vi "lijndetectie.vi"() -> ()   [LabVIEW 2019]
uses:
  <vilib>/Analysis/baseanly.llb/Real Dot Product.vi
  <vilib>/Analysis/NI_AALBase.lvlib
panel:
  out "?":i32
  out "motoren uit (stoppen)":bool
  out "motor links sneller 3":bool
  out "allebei even snel":bool
  out "motor rechts sneller":bool
  in  "input array":dbl[](array[numeric])
  in  "array 2":dbl[](array[numeric])
  out "array gelijk?":string="array gelijk"
  out "array gelijk?":bool[](array[boolean])
  out "true false output 2":bool[](array[boolean])
  out "true false output":bool[](array[boolean])
  out "aantal enen  instant":i32
  out "aantal enen":i32
  in  "array 1":dbl[](array[numeric])
  in  "Numeric 5":dbl
  out "Numeric 4":dbl
  in  "Numeric 2":dbl
  out "output array 2":i32[](array[numeric])
  out "output array":i32[](array[numeric])
  in  "Numeric 3":i32
  out "Numeric":i32
  out "dot product laatste 3 elmenten":dbl format="%.2f"
  out "X * Y":dbl format="%.2f"
  out "som":dbl
  out "x*y":dbl[](array[numeric])
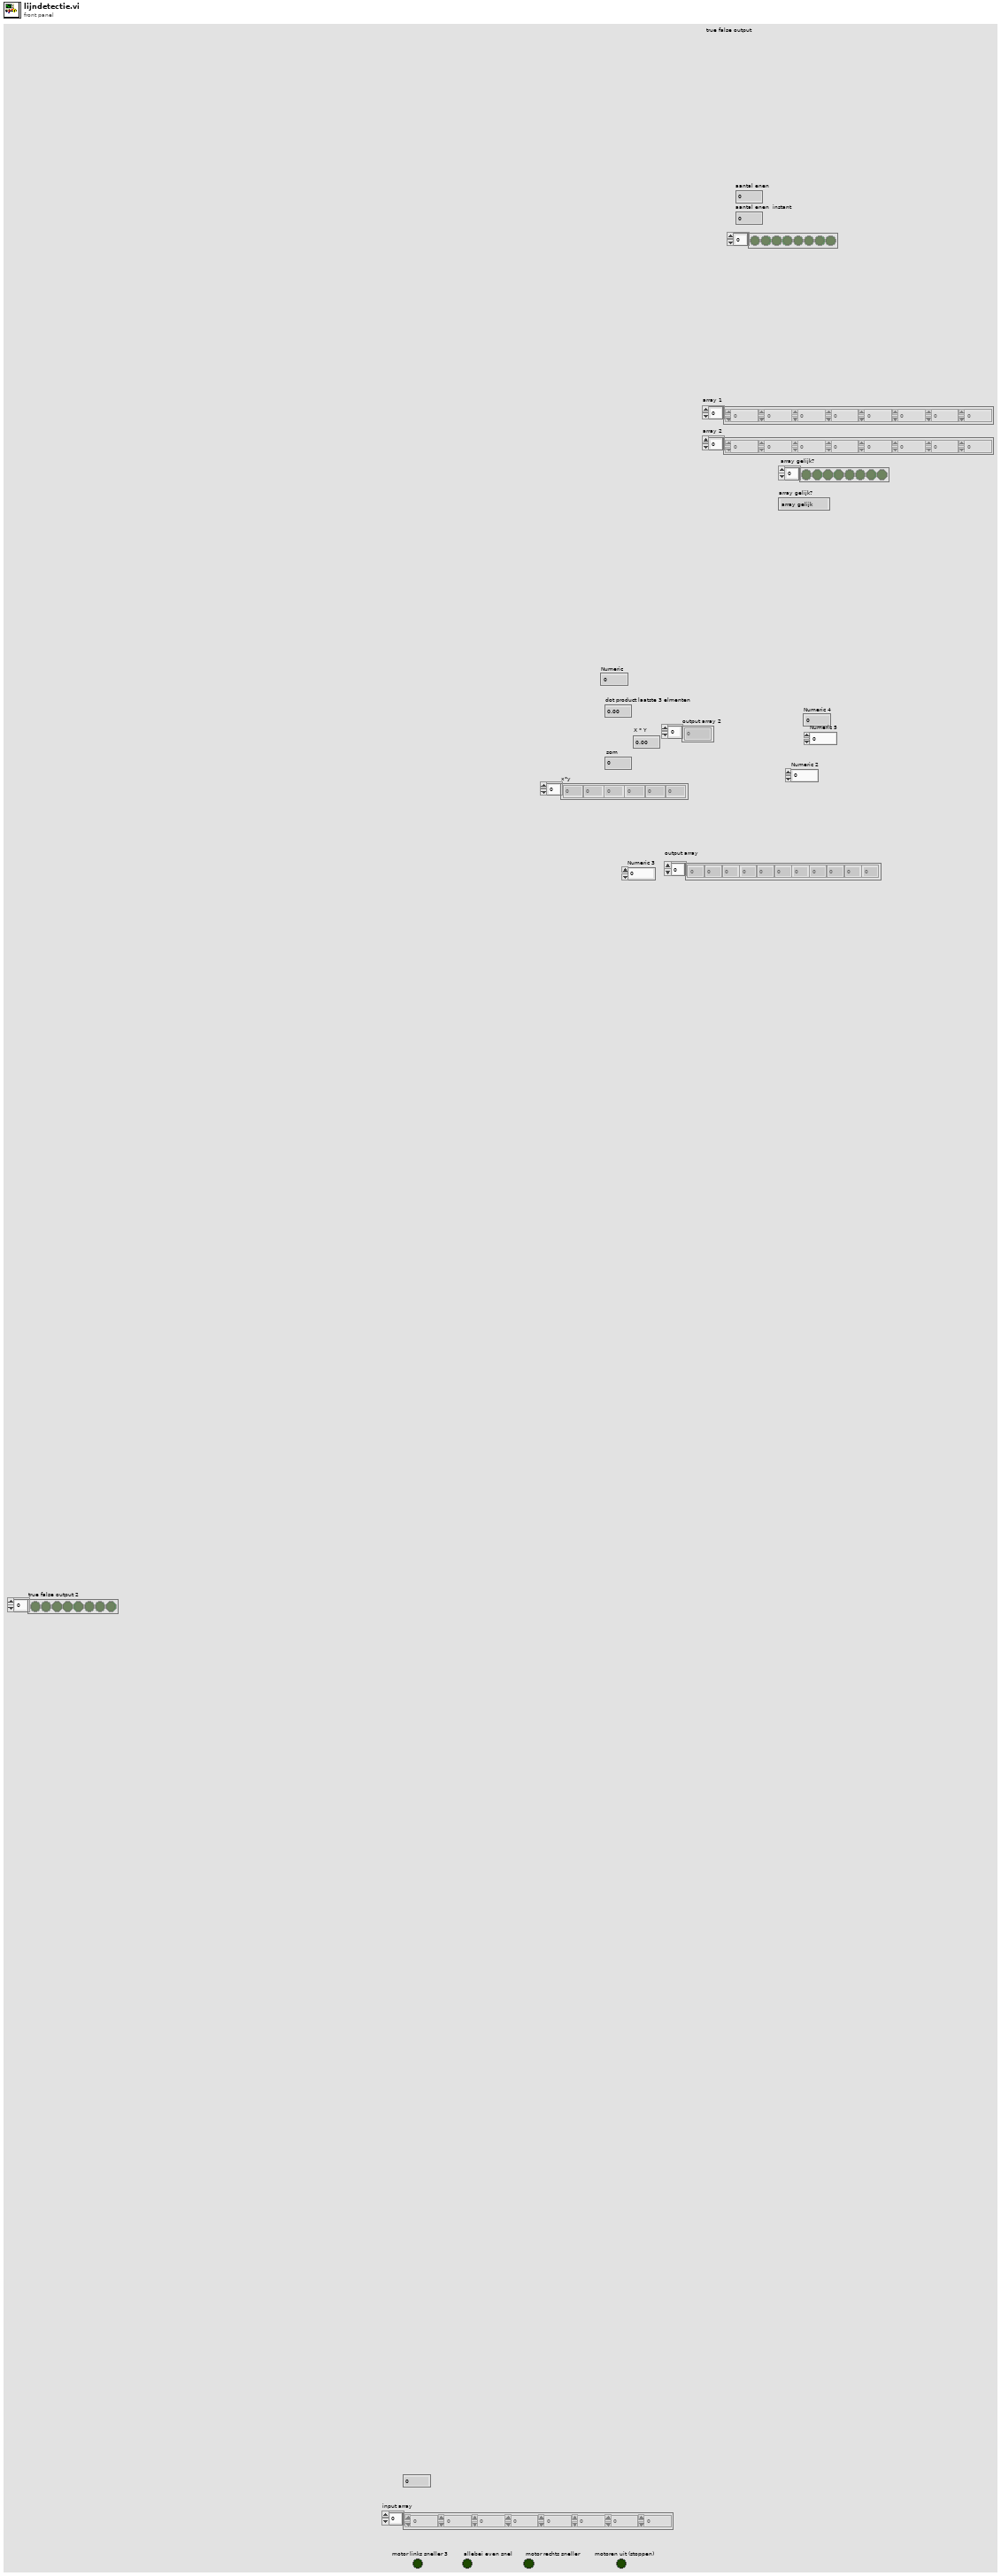
[diagram p1: front panel]
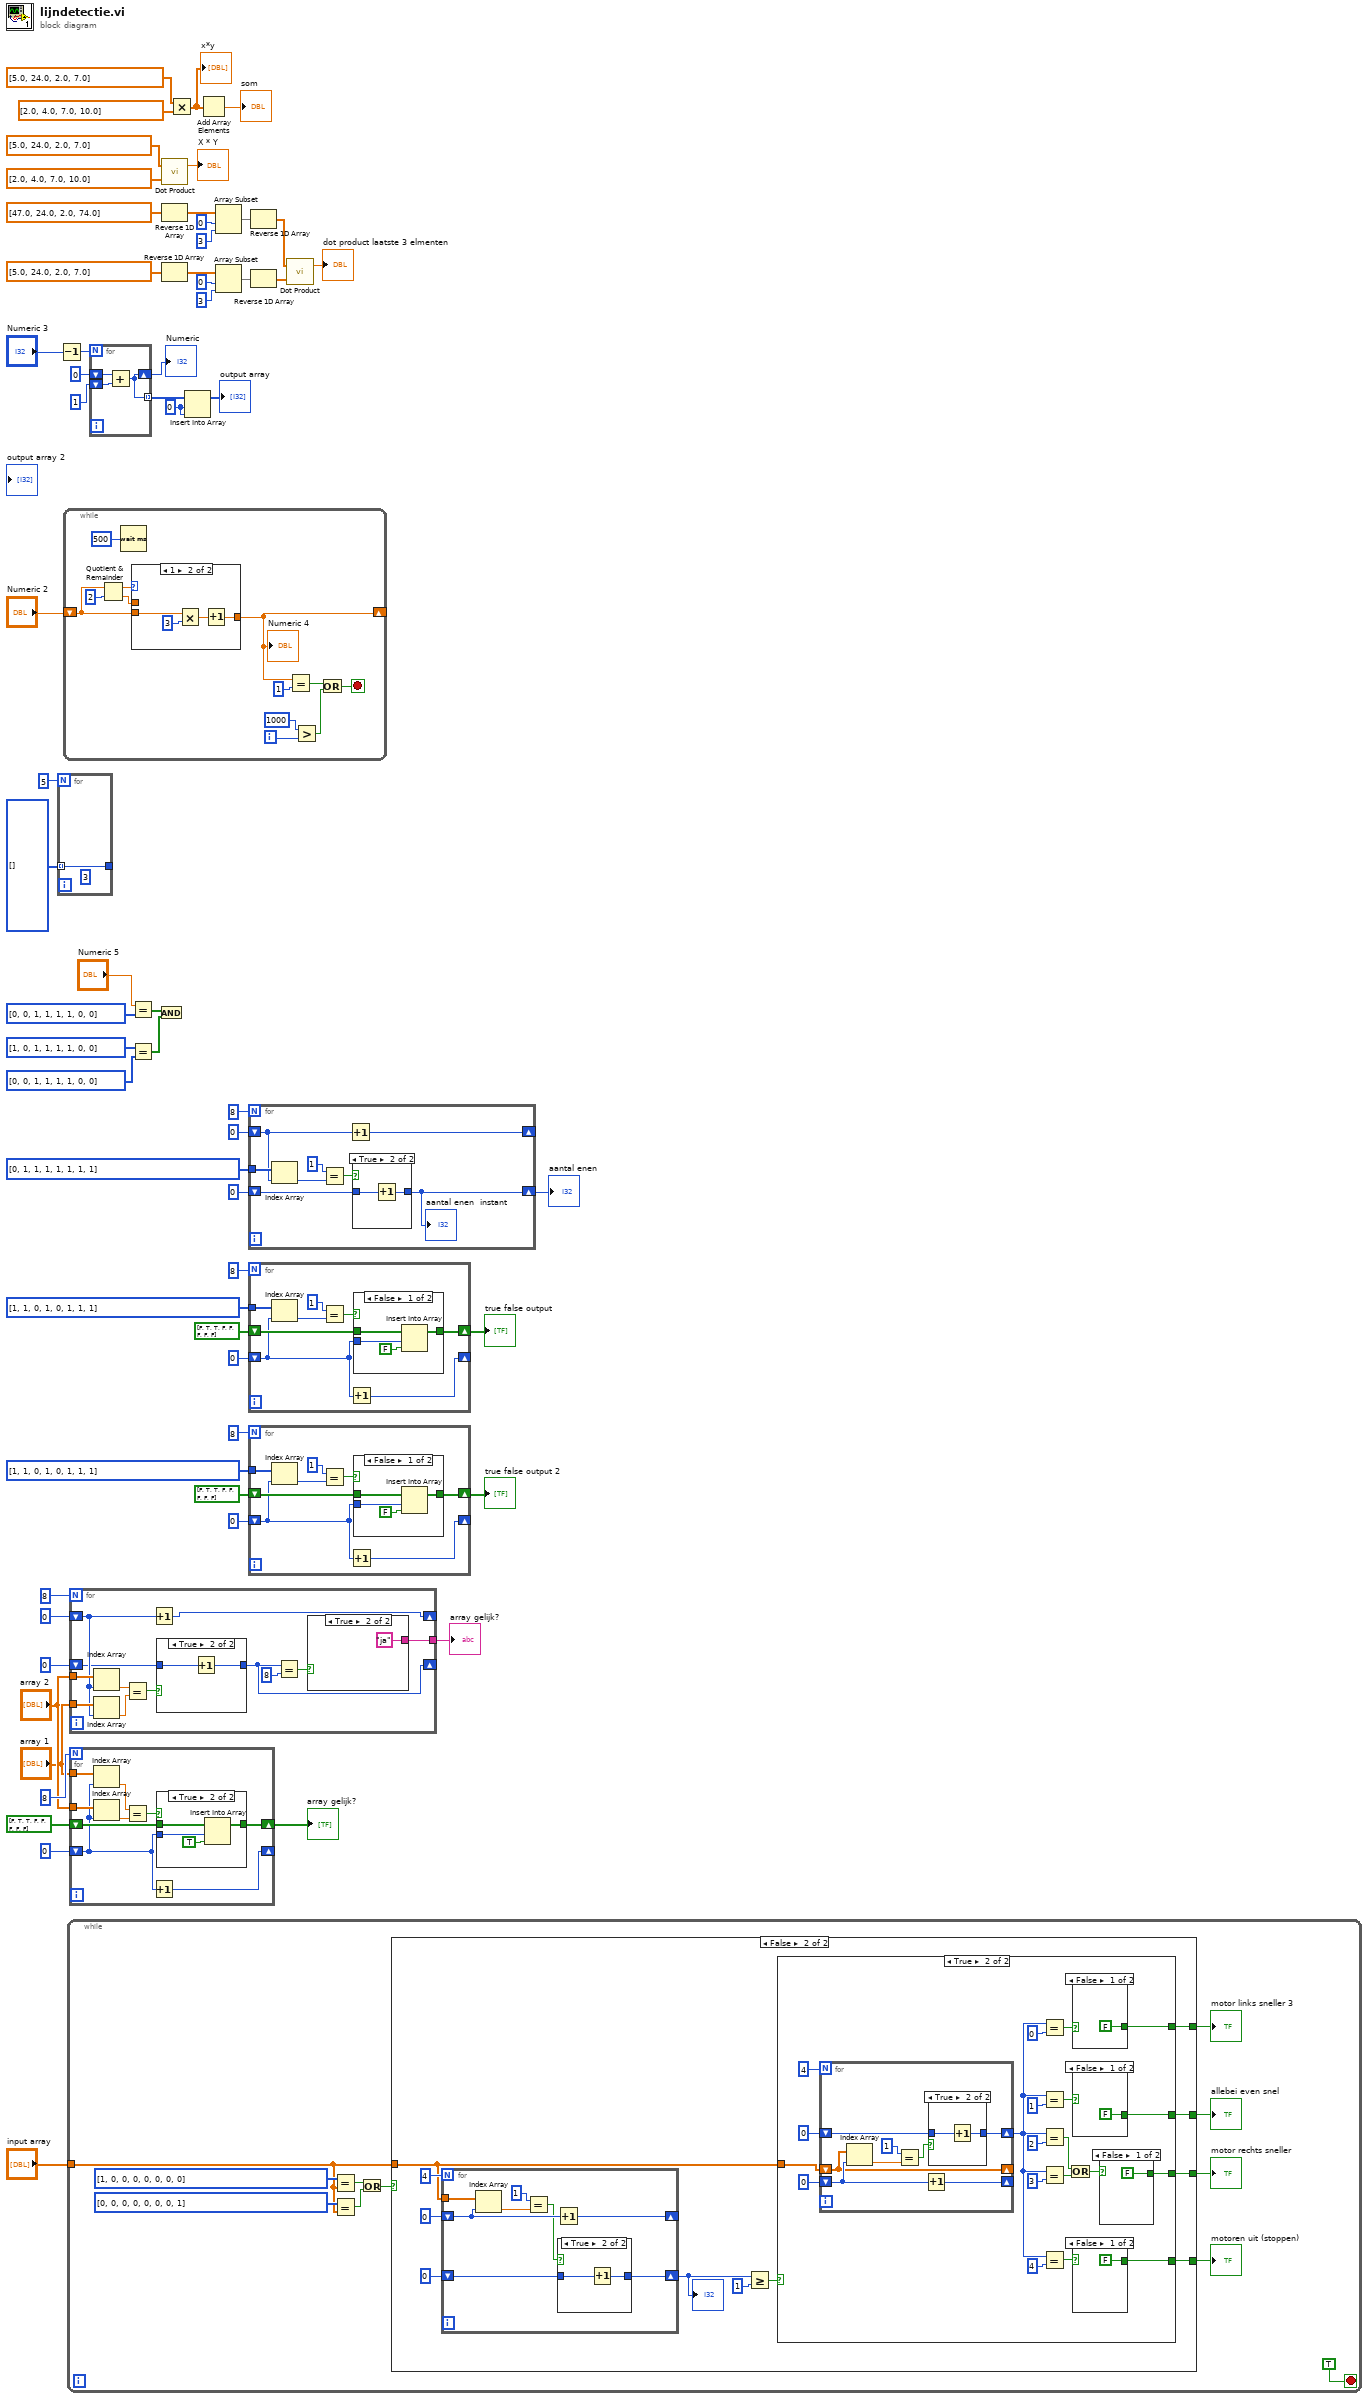
[diagram p0: block diagram]
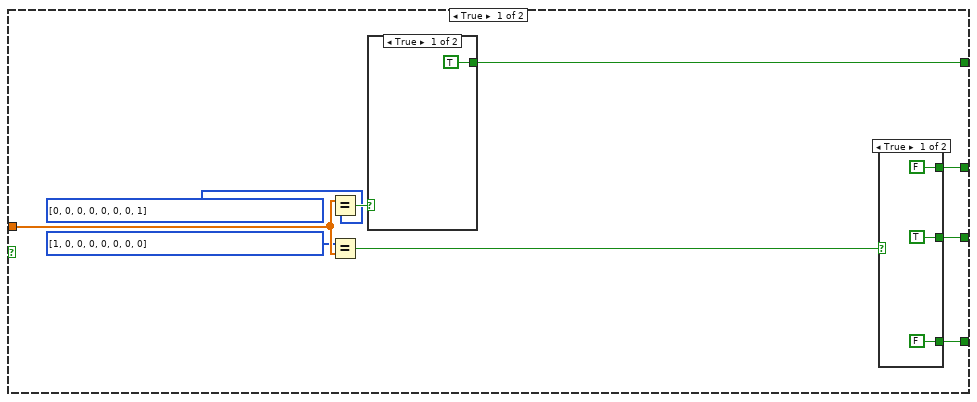
[diagram p2: hidden frame]
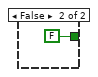
[diagram p3: hidden frame]
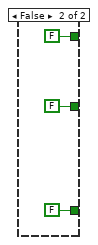
[diagram p4: hidden frame]
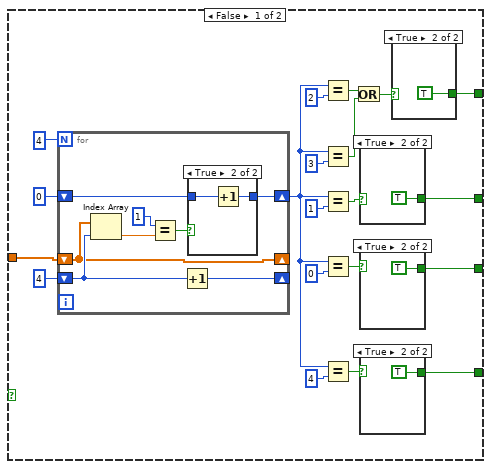
[diagram p6: hidden frame]
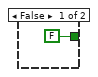
[diagram p7: hidden frame]
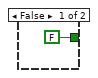
[diagram p8: hidden frame]
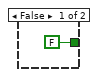
[diagram p9: hidden frame]
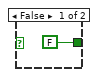
[diagram p10: hidden frame]
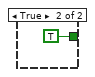
[diagram p12: hidden frame]
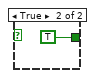
[diagram p13: hidden frame]
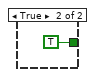
[diagram p14: hidden frame]
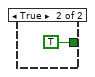
[diagram p15: hidden frame]
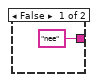
[diagram p17: hidden frame]
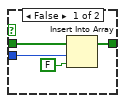
[diagram p19: hidden frame]
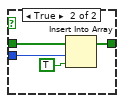
[diagram p20: hidden frame]
diagram:
  w38 = 0
  n1 = for {
    N: 5 -> [_]
    tunnel: i32[] [] -> [w64] mode=indexing
    tunnel: [w64] -> _
    (unwired) 3
  }
  n2 = Decrement(x="Numeric 3") -> (x-1=w39:i32)
  n3 = while {
    shift-right: [w66] -> _
    shift-left: "Numeric 2" -> [w74]
    i -> [w71]
    stop <- w67 stop-if-true
    n4 = Quotient & Remainder(x=w74, y=2) -> (x-y*floor(x/y)=w76:dbl, floor(x/y)=w73:dbl)
    n5 = Wait (ms)(milliseconds to wait=500) -> ()  [unwired: 1 out]
    n6 = case shown="1" w76 {
      tunnel: w74 -> [w78 w82]
      tunnel: w73 -> [_ _]
      tunnel: [w80 w84] -> w66
      frame 0, Default {
        n7 = Multiply(x=w78, y=3) -> (x*y=w79:dbl)
        n8 = Increment(x=w79) -> (x+1=w80:dbl)
      }
      frame 1 {
        n9 = Multiply(x=w82, y=3) -> (x*y=w83:dbl)
        n10 = Increment(x=w83) -> (x+1=w84:dbl)
      }
    }
    "Numeric 4" <- w66
    n11 = Equal?(x=w66, y=1) -> (x = y?=w69:bool)
    n12 = Greater?(x=1000, y=w71) -> (0:w68:bool)
    n13 = Or(x=w69, y=w68) -> (x .or. y?=w67:bool)
  }
  n14 = while {
    tunnel: "input array" -> [w86]
    stop <- TRUE stop-if-true
    n15 = Equal?(x=i32[] [1, 0, 0, 0, 0, 0, 0, 0], y=w86) -> (x = y?=w90:bool)
    n16 = Equal?(x=i32[] [0, 0, 0, 0, 0, 0, 0, 1], y=w86) -> (x = y?=w89:bool)
    n17 = Or(x=w90, y=w89) -> (x .or. y?=w85:bool)
    n18 = case shown="False" w85 {
      tunnel: [w98 w123] -> w94
      tunnel: [w97 w122] -> w93
      tunnel: [w96 w121] -> w92
      tunnel: [w99 w120] -> w91
      tunnel: w86 -> [w103 w113]
      frame True {
        n19 = Equal?(x=w103, y=i32[] [0, 0, 0, 0, 0, 0, 0, 1]) -> (x = y?=w104:bool)
        n20 = Equal?(x=i32[] [1, 0, 0, 0, 0, 0, 0, 0], y=w103) -> (x = y?=w100:bool)
        n21 = case shown="True" w104 {
          tunnel: [TRUE FALSE] -> w99
          frame True {
          }
          frame False {
          }
        }
        n22 = case shown="True" w100 {
          tunnel: [TRUE FALSE] -> w97
          tunnel: [FALSE FALSE] -> w96
          tunnel: [FALSE FALSE] -> w98
          frame True {
          }
          frame False {
          }
        }
      }
      frame False {
        n23 = for {
          N: 4 -> [_]
          tunnel: w113 -> [w131]
          shift-right: [w125] -> _
          shift-left: 0 -> [w130]
          shift-right: [w124] -> w114
          shift-left: 0 -> [w126]
          n24 = Index Array(array=w131, index=w130) -> (element=w129:dbl)
          n25 = Equal?(x=1, y=w129) -> (x = y?=w128:bool)
          n26 = Increment(x=w130) -> (x+1=w125:i32)
          n27 = case shown="True" w128 {
            tunnel: [w132 w134] -> w124
            tunnel: w126 -> [w132 w133]
            frame False {
            }
            frame True {
              n28 = Increment(x=w133) -> (x+1=w134:i32)
            }
          }
        }
        "?" <- w114
        n29 = Greater Or Equal?(x=w114, y=1) -> (x >= y?=w116:bool)
        n30 = case shown="True" w116 {
          tunnel: [w142 w183] -> w123
          tunnel: [w143 w182] -> w122
          tunnel: [w144 w181] -> w121
          tunnel: [w145 w180] -> w120
          tunnel: w113 -> [w141 w179]
          frame False {
            n31 = for {
              N: 4 -> [_]
              shift-right: [w169] -> _
              shift-left: 4 -> [w170]
              shift-right: [w165] -> w138
              shift-left: 0 -> [w166]
              shift-right: [w163] -> _
              shift-left: w141 -> [w163]
              n32 = Index Array(array=w163, index=w170) -> (element=w164:dbl)
              n33 = Equal?(x=1, y=w164) -> (x = y?=w168:bool)
              n34 = Increment(x=w170) -> (x+1=w169:i32)
              n35 = case shown="True" w168 {
                tunnel: [w171 w173] -> w165
                tunnel: w166 -> [w171 w172]
                frame False {
                }
                frame True {
                  n36 = Increment(x=w172) -> (x+1=w173:i32)
                }
              }
            }
            n37 = Equal?(x=w138, y=2) -> (x = y?=w136:bool)
            n38 = Equal?(x=w138, y=3) -> (x = y?=w135:bool)
            n39 = Equal?(x=w138, y=1) -> (x = y?=w148:bool)
            n40 = Equal?(x=w138, y=0) -> (x = y?=w147:bool)
            n41 = Equal?(x=w138, y=4) -> (x = y?=w146:bool)
            n42 = Or(x=w136, y=w135) -> (x .or. y?=w137:bool)
            n43 = case shown="True" w148 {
              tunnel: [FALSE ("Boolean 2") TRUE] -> w144
              frame False {
              }
              frame True {
              }
            }
            n44 = case shown="True" w147 {
              tunnel: [FALSE ("Boolean 2") TRUE] -> w143
              frame False {
              }
              frame True {
              }
            }
            n45 = case shown="True" w146 {
              tunnel: [FALSE ("Boolean 2") TRUE] -> w142
              frame False {
              }
              frame True {
              }
            }
            n46 = case shown="True" w137 {
              tunnel: [FALSE ("Boolean 2") TRUE] -> w145
              frame False {
              }
              frame True {
              }
            }
          }
          frame True {
            n47 = for {
              N: 4 -> [_]
              shift-right: [w208] -> _
              shift-left: 0 -> [w209]
              shift-right: [w204] -> w176
              shift-left: 0 -> [w205]
              shift-right: [w202] -> _
              shift-left: w179 -> [w202]
              n48 = Index Array(array=w202, index=w209) -> (element=w203:dbl)
              n49 = Equal?(x=1, y=w203) -> (x = y?=w207:bool)
              n50 = Increment(x=w209) -> (x+1=w208:i32)
              n51 = case shown="True" w207 {
                tunnel: [w210 w212] -> w204
                tunnel: w205 -> [w210 w211]
                frame False {
                }
                frame True {
                  n52 = Increment(x=w211) -> (x+1=w212:i32)
                }
              }
            }
            n53 = Equal?(x=w176, y=0) -> (x = y?=w186:bool)
            n54 = Equal?(x=w176, y=1) -> (x = y?=w185:bool)
            n55 = Equal?(x=w176, y=2) -> (x = y?=w174:bool)
            n56 = Equal?(x=w176, y=3) -> (x = y?=w177:bool)
            n57 = Equal?(x=w176, y=4) -> (x = y?=w184:bool)
            n58 = Or(x=w174, y=w177) -> (x .or. y?=w175:bool)
            n59 = case shown="False" w186 {
              tunnel: [FALSE ("Boolean 2") TRUE ("Boolean 2")] -> w180
              frame False {
              }
              frame True {
              }
            }
            n60 = case shown="False" w185 {
              tunnel: [FALSE ("Boolean 2") TRUE ("Boolean 2")] -> w181
              frame False {
              }
              frame True {
              }
            }
            n61 = case shown="False" w184 {
              tunnel: [FALSE ("Boolean 2") TRUE ("Boolean 2")] -> w183
              frame False {
              }
              frame True {
              }
            }
            n62 = case shown="False" w175 {
              tunnel: [FALSE ("Boolean 2") TRUE ("Boolean 2")] -> w182
              frame False {
              }
              frame True {
              }
            }
          }
        }
      }
    }
    "motor rechts sneller" <- w93
    "allebei even snel" <- w92
    "motor links sneller 3" <- w91
    "motoren uit (stoppen)" <- w94
  }
  n63 = for {
    N: 8 -> [_]
    shift-right: [w224] -> _
    shift-left: 0 -> [w218]
    tunnel: "array 2" -> [w223]
    tunnel: "array 1" -> [w222]
    shift-right: [w215] -> _
    shift-left: 0 -> [w217]
    tunnel: [w213] -> w4
    n64 = Index Array(array=w223, index=w218) -> (element=w221:dbl)
    n65 = Index Array(array=w222, index=w218) -> (element=w220:dbl)
    n66 = Equal?(x=w221, y=w220) -> (x = y?=w219:bool)
    n67 = Increment(x=w218) -> (x+1=w224:i32)
    n68 = case shown="True" w219 {
      tunnel: w217 -> [w227 w229]
      tunnel: [w227 w228] -> w215
      frame False {
      }
      frame True {
        n69 = Increment(x=w229) -> (x+1=w228:i32)
      }
    }
    n70 = Equal?(x=w215, y=8) -> (x = y?=w216:bool)
    n71 = case shown="True" w216 {
      tunnel: ["nee" "ja"] -> w213
      frame False {
      }
      frame True {
      }
    }
  }
  "array gelijk?" <- w4
  n72 = for {
    N: 8 -> [_]
    shift-right: [w238] -> _
    shift-left: 0 -> [w231]
    shift-right: [w230] -> w8
    shift-left: bool[] [FALSE, TRUE, TRUE, FALSE, FALSE, FALSE, FALSE, FALSE] -> [w232]
    tunnel: "array 1" -> [w237]
    tunnel: "array 2" -> [w236]
    n73 = Index Array(array=w237, index=w231) -> (element=w235:dbl)
    n74 = Index Array(array=w236, index=w231) -> (element=w234:dbl)
    n75 = Equal?(x=w235, y=w234) -> (x = y?=w233:bool)
    n76 = Increment(x=w231) -> (x+1=w238:i32)
    n77 = case shown="True" w233 {
      tunnel: w232 -> [w241 w245]
      tunnel: w231 -> [w240 w244]
      tunnel: [w239 w243] -> w230
      frame False {
        n78 = Insert Into Array(array=w241, index=w240, new element=FALSE) -> (w239:bool[])
      }
      frame True {
        n79 = Insert Into Array(array=w245, index=w244, new element=TRUE) -> (w243:bool[])
      }
    }
  }
  "array gelijk?" <- w8
  n80 = for {
    N: w39 -> [_]
    shift-right: [w247] -> w42
    shift-left: 0 -> [w249]
    shift-left: 1 -> [w248]
    tunnel: [w247] -> w37 mode=indexing
    n81 = Add(x=w249, y=w248) -> (x+y=w247:i32)
  }
  "Numeric" <- w42
  n82 = Equal?(x="Numeric 5", y=i32[] [0, 0, 1, 1, 1, 1, 0, 0]) -> (x = y?=w28:bool[])
  n83 = Equal?(x=i32[] [1, 0, 1, 1, 1, 1, 0, 0], y=i32[] [0, 0, 1, 1, 1, 1, 0, 0]) -> (x = y?=w27:bool[])
  n84 = And(x=w28, y=w27) -> ()  [unwired: 1 out]
  n85 = Reverse 1D Array(array=dbl[] [47.0, 24.0, 2.0, 74.0]) -> (reversed array=w53:dbl[])
  n86 = Reverse 1D Array(array=dbl[] [5.0, 24.0, 2.0, 7.0]) -> (reversed array=w49:dbl[])
  n87 = call-poly <vilib>:"Dot Product.vi"("Y Vector"=dbl[] [2.0, 4.0, 7.0, 10.0], "X Vector"=dbl[] [5.0, 24.0, 2.0, 7.0]) -> ("X * Y"=→"X * Y":dbl)  [unwired: 1 out]
  n88 = Multiply(x=dbl[] [5.0, 24.0, 2.0, 7.0], y=dbl[] [2.0, 4.0, 7.0, 10.0]) -> (x*y=w62:dbl[])
  "x*y" <- w62
  n89 = Insert Into Array(array=w37, index=w38, new element=w38) -> (→"output array":i32[])
  n90 = Add Array Elements(numeric array=w62) -> (sum=→"som":dbl)
  n91 = Array Subset(array=w53, index=0, length=3) -> (w52:dbl[])
  n92 = Array Subset(array=w49, index=0, length=3) -> (w48:dbl[])
  n93 = for {
    N: 8 -> [_]
    tunnel: i32[] [0, 1, 1, 1, 1, 1, 1, 1] -> [w257]
    shift-right: [w255] -> _
    shift-left: 0 -> [w256]
    shift-right: [w250] -> w22
    shift-left: 0 -> [w251]
    n94 = Index Array(array=w257, index=w256) -> (element=w254:i32)
    n95 = Equal?(x=1, y=w254) -> (x = y?=w253:bool)
    n96 = Increment(x=w256) -> (x+1=w255:i32)
    n97 = case shown="True" w253 {
      tunnel: [w258 w260] -> w250
      tunnel: w251 -> [w258 w259]
      frame False {
      }
      frame True {
        n98 = Increment(x=w259) -> (x+1=w260:i32)
      }
    }
    "aantal enen  instant" <- w250
  }
  "aantal enen" <- w22
  n99 = for {
    N: 8 -> [_]
    tunnel: i32[] [1, 1, 0, 1, 0, 1, 1, 1] -> [w268]
    shift-right: [w267] -> _
    shift-left: 0 -> [w263]
    shift-right: [w262] -> w17
    shift-left: bool[] [FALSE, TRUE, TRUE, FALSE, FALSE, FALSE, FALSE, FALSE] -> [w264]
    n100 = Index Array(array=w268, index=w263) -> (element=w266:i32)
    n101 = Equal?(x=1, y=w266) -> (x = y?=w261:bool)
    n102 = Increment(x=w263) -> (x+1=w267:i32)
    n103 = case shown="False" w261 {
      tunnel: [w269 w275] -> w262
      tunnel: w264 -> [w272 w274]
      tunnel: w263 -> [w271 w273]
      frame False {
        n104 = Insert Into Array(array=w272, index=w271, new element=FALSE) -> (w269:bool[])
      }
      frame True {
        n105 = Insert Into Array(array=w274, index=w273, new element=TRUE) -> (w275:bool[])
      }
    }
  }
  "true false output" <- w17
  n106 = for {
    N: 8 -> [_]
    tunnel: i32[] [1, 1, 0, 1, 0, 1, 1, 1] -> [w284]
    shift-right: [w283] -> _
    shift-left: 0 -> [w279]
    shift-right: [w278] -> w12
    shift-left: bool[] [FALSE, TRUE, TRUE, FALSE, FALSE, FALSE, FALSE, FALSE] -> [w280]
    n107 = Index Array(array=w284, index=w279) -> (element=w282:i32)
    n108 = Equal?(x=1, y=w282) -> (x = y?=w277:bool)
    n109 = Increment(x=w279) -> (x+1=w283:i32)
    n110 = case shown="False" w277 {
      tunnel: [w285 w291] -> w278
      tunnel: w280 -> [w288 w290]
      tunnel: w279 -> [w287 w289]
      frame False {
        n111 = Insert Into Array(array=w288, index=w287, new element=FALSE) -> (w285:bool[])
      }
      frame True {
        n112 = Insert Into Array(array=w290, index=w289, new element=TRUE) -> (w291:bool[])
      }
    }
  }
  "true false output 2" <- w12
  n113 = Reverse 1D Array(array=w52) -> (reversed array=w45:dbl[])
  n114 = Reverse 1D Array(array=w48) -> (reversed array=w44:dbl[])
  n115 = call-poly <vilib>:"Dot Product.vi"("Y Vector"=w44, "X Vector"=w45) -> ("X * Y"=→"dot product laatste 3 elmenten":dbl)  [unwired: 1 out]
